vi "Obtain Broadcast Events.vi"(8 "error in (no error)":errorcluster, 10 "Create New? (F)":bool) -> (0 "error out":errorcluster, 2 "TDS1002 Oscilloscope Broadcast Events":T1)   [LabVIEW 2020, in "TDS1002 Oscilloscope.lvlib"]
doc: "This VI Obtains/Creates the Broadcast events that will be used for other modules to register to receive messages from the module that owns this VI.\n\n<b>NOTE</b>: The contents of this VI are automatically generated and modified by the <b>Tools > Delacor > DQMH</b> utilities. Consider using those utilities instead of making your own modifications to this VI.\n_____\nBased on DQMH Project Template 6.1.0.94.\n____\nPantherLAB Templates 1.0.0.1\nCopyright (c) 2022, PantherLAB\n____\nPantherLAB Templates 1.0.0.5\nCopyright (c) 2022, PantherLAB"
uses:
  TDS1002 Oscilloscope.lvlib
  Broadcast Events--cluster.ctl
  Did Init Argument--cluster.ctl
  Status Updated Argument--cluster.ctl
  Error Reported Argument--cluster.ctl
  Stop Argument--cluster.ctl
  Get Module Execution Status Argument--cluster.ctl
  Helper Loop Status Updated Argument--cluster.ctl
  Helper Loop Status--enum.ctl
  Device connected Argument--cluster.ctl
  Device disconnected Argument--cluster.ctl
  Data acquired Argument--cluster.ctl
  Configuration applied Argument--cluster.ctl
panel:
  # "NOTE: The contents of this VI are automatically generated and modified by the Tools > Delacor > DQMH utilities. Consider using those utilities instead of making your own modifications to this VI."
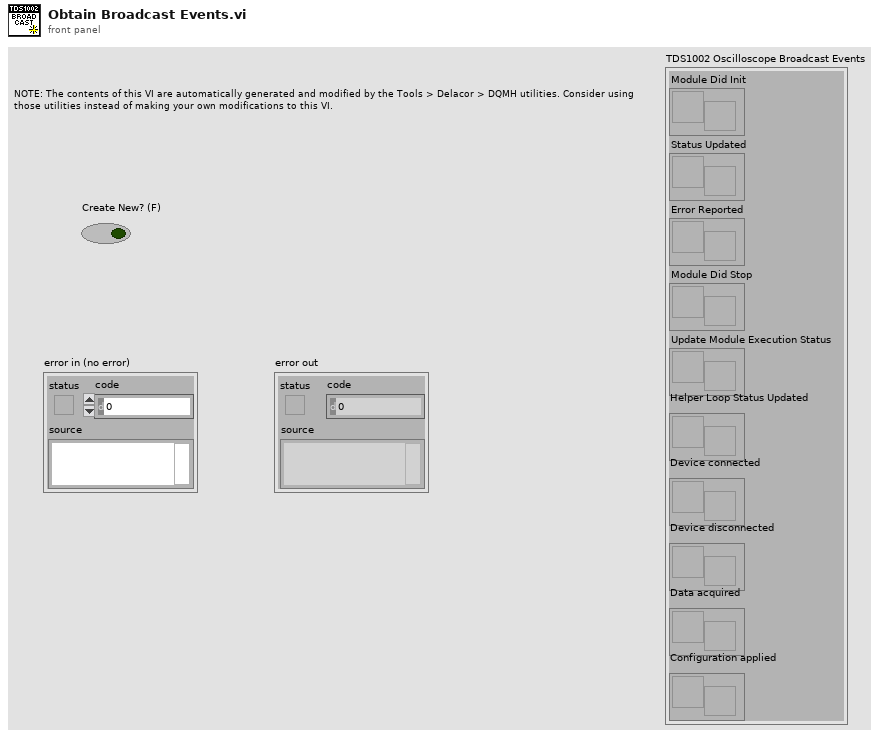
[diagram p1: front panel]
types:
  T1 = typedef "TDS1002 Oscilloscope.lvlib/Broadcast Events--cluster.ctl" = cluster{"Module Did Init":refnum<user-event>, "Status Updated":refnum<user-event>, "Error Reported":refnum<user-event>, "Module Did Stop":refnum<user-event>, "Update Module Execution Status":refnum<user-event>, "Helper Loop Status Updated":refnum<user-event>, "Device connected":refnum<user-event>, "Device disconnected":refnum<user-event>, "Data acquired":refnum<user-event>, "Configuration applied":refnum<user-event>}
  T2 = typedef "TDS1002 Oscilloscope.lvlib/Configuration applied Argument--cluster.ctl" = cluster{"Module ID":i32, "Boolean":bool}
  T3 = typedef "TDS1002 Oscilloscope.lvlib/Data acquired Argument--cluster.ctl" = cluster{"Module ID":i32, "Waveform":waveform(dbl)}
  T4 = typedef "TDS1002 Oscilloscope.lvlib/Device disconnected Argument--cluster.ctl" = cluster{"Module ID":i32, "Boolean":bool}
  T5 = typedef "TDS1002 Oscilloscope.lvlib/Device connected Argument--cluster.ctl" = cluster{"Module ID":i32, "Boolean":bool}
  T6 = typedef "TDS1002 Oscilloscope.lvlib/Helper Loop Status Updated Argument--cluster.ctl" = cluster{"Module ID":i32, "Helper Loop Status":T7}
  T7 = typedef "TDS1002 Oscilloscope.lvlib/Helper Loop Status--enum.ctl" = enum16{"Awake", "Asleep"}
  T8 = typedef "TDS1002 Oscilloscope.lvlib/Get Module Execution Status Argument--cluster.ctl" = cluster{"Module ID":i32, "Running?":bool}
  T9 = typedef "TDS1002 Oscilloscope.lvlib/Stop Argument--cluster.ctl" = cluster{"Module ID":i32, "Origin":string, "Exit via Stop Module Req?":bool, "Wait for Module to stop?":bool}
  T10 = typedef "TDS1002 Oscilloscope.lvlib/Error Reported Argument--cluster.ctl" = cluster{"Error":errorcluster, "Additional Information":string, "Module ID":i32, "Module Name":string}
  T11 = typedef "TDS1002 Oscilloscope.lvlib/Status Updated Argument--cluster.ctl" = cluster{"Status":string, "Module ID":i32}
  T12 = typedef "TDS1002 Oscilloscope.lvlib/Did Init Argument--cluster.ctl" = cluster{"Init?":bool, "Info":string, "Module ID":i32}
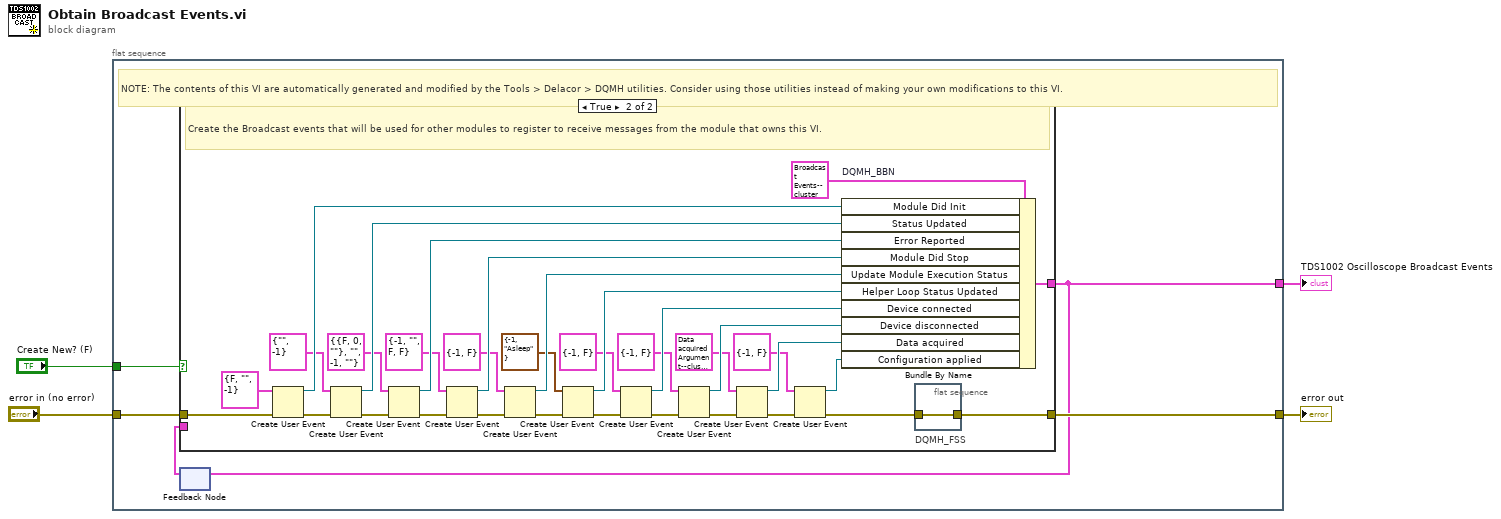
[diagram p0: block diagram]
diagram:
  n1 = flat-sequence {
    tunnel: [w9] -> w4
    tunnel: "error in (no error)" -> [w8]
    tunnel: [w6] -> w2
    tunnel: "Create New? (F)" -> [w5]
    frame #0 {
      # "NOTE: The contents of this VI are automatically generated and modified by the Tools > Delacor > DQMH utilities. Consider using those utilities instead of making your own modifications to this VI."
      n2 = feedback #1() -> (w7:T1)  [unwired: 1 in]
      n3 = case shown="True" w5 {
        tunnel: [w10 w30] -> w9
        tunnel: w8 -> [w10 w45]
        tunnel: [w11 w42] -> w6
        tunnel: w7 -> [w11 _]
        frame False {
          # "Obtain the Broadcast events that were created in a previous call to this VI."
        }
        frame True {
          # "Create the Broadcast events that will be used for other modules to register to receive messages from the module that owns this VI."
          n4 = Create User Event(user event datatype=T12 {"Init?"=FALSE, "Info"="", "Module ID"=-1} ("Did Init Argument"), error in=w45) -> (user event=w43:refnum<user-event>, error out=w40:errorcluster)
          n5 = Create User Event(user event datatype=T11 {"Status"="", "Module ID"=-1} ("Status Updated Argument"), error in=w40) -> (user event=w37:refnum<user-event>, error out=w39:errorcluster)
          n6 = Create User Event(user event datatype=T10 {"Error"={"status"=FALSE, "code"=0, "source"=""}, "Additional Information"="", "Module ID"=-1, "Module Name"=""} ("Error Reported Argument"), error in=w39) -> (user event=w34:refnum<user-event>, error out=w36:errorcluster)
          n7 = Create User Event(user event datatype=T9 {"Module ID"=-1, "Origin"="", "Exit via Stop Module Req?"=FALSE, "Wait for Module to stop?"=FALSE} ("Stop Argument"), error in=w36) -> (user event=w32:refnum<user-event>, error out=w31:errorcluster)
          n8 = Create User Event(user event datatype=T8 {"Module ID"=-1, "Running?"=FALSE} ("Get Module Execution Status Argument"), error in=w31) -> (user event=w28:refnum<user-event>, error out=w29:errorcluster)
          n9 = Create User Event(user event datatype=T6 {"Module ID"=-1, "Helper Loop Status"=enum."Asleep"} ("Helper Loop Status Updated Argument"), error in=w29) -> (user event=w25:refnum<user-event>, error out=w26:errorcluster)
          n10 = Create User Event(user event datatype=T5 {"Module ID"=-1, "Boolean"=FALSE} ("Device connected Argument"), error in=w26) -> (user event=w22:refnum<user-event>, error out=w23:errorcluster)
          n11 = Create User Event(user event datatype=T4 {"Module ID"=-1, "Boolean"=FALSE} ("Device disconnected Argument"), error in=w23) -> (user event=w19:refnum<user-event>, error out=w20:errorcluster)
          n12 = Create User Event(user event datatype=T3 {"Module ID"=-1, "Waveform"={"t0"=timestamp(0 s since 1904-01-01), "dt"=1.0, "Y"=[]}} ("Data acquired Argument"), error in=w20) -> (user event=w16:refnum<user-event>, error out=w17:errorcluster)
          n13 = Create User Event(user event datatype=T2 {"Module ID"=-1, "Boolean"=FALSE} ("Configuration applied Argument"), error in=w17) -> (user event=w13:refnum<user-event>, error out=w14:errorcluster)
          n14 = Bundle By Name "DQMH_BBN"(cluster=T1 {"Module Did Init"=refnum, "Status Updated"=refnum, "Error Reported"=refnum, "Module Did Stop"=refnum, "Update Module Execution Status"=refnum, "Helper Loop Status Updated"=refnum, "Device connected"=refnum, "Device disconnected"=refnum, "Data acquired"=refnum, "Configuration applied"=refnum} ("output cluster"), "Module Did Init"=w43, "Status Updated"=w37, "Error Reported"=w34, "Module Did Stop"=w32, "Update Module Execution Status"=w28, "Helper Loop Status Updated"=w25, "Device connected"=w22, "Device disconnected"=w19, "Data acquired"=w16, "Configuration applied"=w13) -> (w42:T1)
          n15 = flat-sequence "DQMH_FSS" {
            tunnel: w14 -> [w46]
            tunnel: [w46] -> w30
            frame #0 {
            }
          }
        }
      }
      n16 = feedback-in #1(w6) -> ()
    }
  }
  "TDS1002 Oscilloscope Broadcast Events" <- w2
  "error out" <- w4
